vi "Handle Last Ack Core.vi"(4 "error in (no error)":errorcluster, 6 "Last Ack":refnum<class "Last Ack.lvclass">, 7 "Hotel Management Tool Model in":refnum<class "Hotel Management Tool Model.lvclass">) -> (0 "error out":errorcluster, 3 "Hotel Management Tool Model out":refnum<class "Hotel Management Tool Model.lvclass">)   [LabVIEW 2023, in "Hotel Management Tool Model.lvlib" / "Hotel Management Tool Model.lvclass"]
doc: "(<B>Filename</B>: Actor Framework.lvlib:Actor.lvclass:Handle Last Ack Core.vi)\n\nDefines how the caller actor responds to the Last Ack message from a nested actor. The Last Ack message is the final message a nested actor sends to its caller before it shuts down. The message contains information about the final state of the nested actor.\n\nBy default, this method does nothing except return any error the nested actor sent. A descendant class may override this method to define behavior."
uses:
  Hotel Management Tool Model.lvclass
  Hotel Management Tool Model.lvclass/Hotel Management Tool Model.ctl
  <vilib>/ActorFramework/LastAck/Last Ack.lvclass
  Model Base/Model Base/Model Base.lvclass
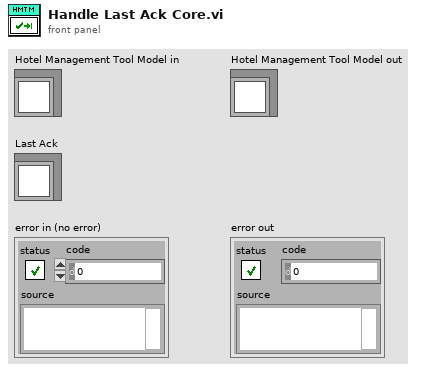
[diagram p1: front panel]
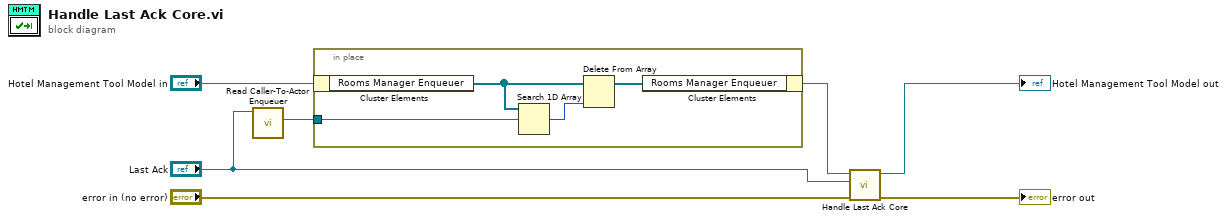
[diagram p0: block diagram]
diagram:
  n1 = call <vilib>:"Read Caller-To-Actor Enqueuer.vi"("Last Ack"="Last Ack") -> ("Caller-to-Actor Enqueuer"=w1:refnum<class "Message Enqueuer.lvclass">)  [unwired: 10 in]
  n2 = in-place {
    in-place-border: w1 -> [w9]
    n3 = in-place-cluster #1("Hotel Management Tool Model in") -> ("Rooms Manager Enqueuer"=w10:refnum<class "Message Enqueuer.lvclass">[])
    n4 = Search 1D Array(1D array=w10, element=w9) -> (index of element=w8:i32)  [unwired: 1 in]
    n5 = Delete From Array(array=w10, index=w8) -> (array with subset deleted=w11:refnum<class "Message Enqueuer.lvclass">[])  [unwired: 1 in, 1 out]
    n6 = in-place-cluster #1("Rooms Manager Enqueuer"=w11) -> (w2:refnum<class "Hotel Management Tool Model.lvclass">)
  }
  n7 = call-parent "Handle Last Ack Core.vi"("error in (no error)"="error in (no error)", "Last Ack"="Last Ack", "Actor in"=w2) -> ("error out"=→"error out":errorcluster, "Actor out"=→"Hotel Management Tool Model out":refnum<class "Hotel Management Tool Model.lvclass">)  [unwired: 3 in]
